vi "Add PV (NT Enum (Enum)).vi"(6 "initial timestamp":timestamp, 7 "PV name":string, 8 "error in (no error)":errorcluster, 10 "initial value":variant, 11 "Server in":refnum<class "Server.lvclass">) -> (0 "error out":errorcluster, 2 "value out":variant, 3 "Server out":refnum<class "Server.lvclass">, 4 "timestamp out":timestamp)   [LabVIEW 2020, in "PV Access.lvlib" / "PVA Server.lvlib" / "Server.lvclass"]
uses:
  Server.lvclass
  PV Data/NT Enum/NT Enum.lvclass
  C:/Users/eyw68381/source/repos/pvaccess-labview/labview/source/PV Data/NT Base/NT Base.lvclass
  <vilib>/Utility/error.llb/Error Cluster From Error Code.vi
  <vilib>/ErrorRing/Error Ring.xnode
  Source/Source.lvclass
  PV Data/PV Data.lvlib
  <userlib>/_OpenG.lib/lvdata/lvdata.llb/openg_variant.lvlib
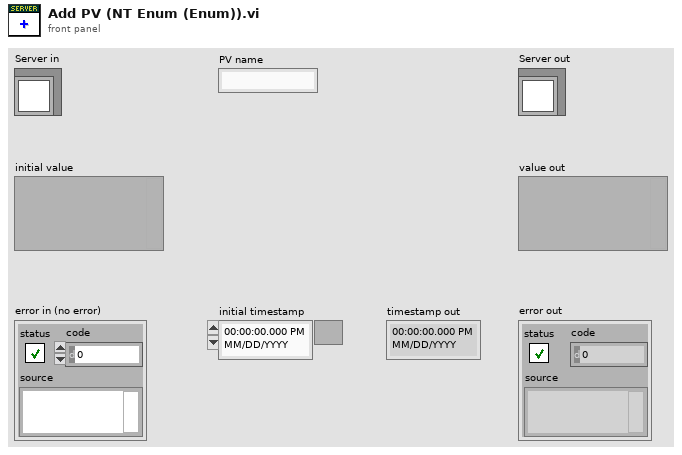
[diagram p1: front panel]
types:
  T1 = typedef "openg_variant.lvlib/Type Descriptor Enumeration__ogtk.ctl" = enum8{"<Null>", "I8", "I16", "I32", "I64", "U8", "U16", "U32", "U64", "SGL", "DBL", "EXT", "CSG", "CDB", "CXT", "0x0F", "0x10", "0x11", "0x12", "0x13", "0x14", "Enum U8", "Enum U16", "Enum U32", "Enum U64", "SGL PQ", "DBL PQ", "EXT PQ", "CSG PQ", "CDB PQ", "CXT PQ", "0x1F", "0x20", "Boolean", "0x22", "0x23", "0x24", "0x25", "0x26", "0x27", "0x28", "0x29", "0x2A", "0x2B", "0x2C", "0x2D", "0x2E", "0x2F", "String", "0x31", "Path", "Pict", "0x34", "0x35", "0x36", "DAQ", "0x38", "0x39", "0x3A", "0x3B", "0x3C", "0x3D", "0x3E", "0x3F", "Array", "0x41", "0x42", "0x43", "0x44", "0x45", "0x46", "0x47", "0x48", "0x49", "0x4A", "0x4B", "0x4C", "0x4D", "0x4E", "0x4F", "Cluster", "0x51", "0x52", "Variant", "Waveform", "0x55", "0x56", "0x57", "0x58", "0x59", "0x5A", "0x5B", "0x5C", "0x5D", "0x5E", "Fixed Point", "0x60", "0x61", "0x62", "0x63", "0x64", "0x65", "0x66", "0x67", "0x68", "0x69", "0x6A", "0x6B", "0x6C", "0x6D", "0x6E", "0x6F", "Refnum", "0x71", "0x72", "Set Collection", "Map Collection"}
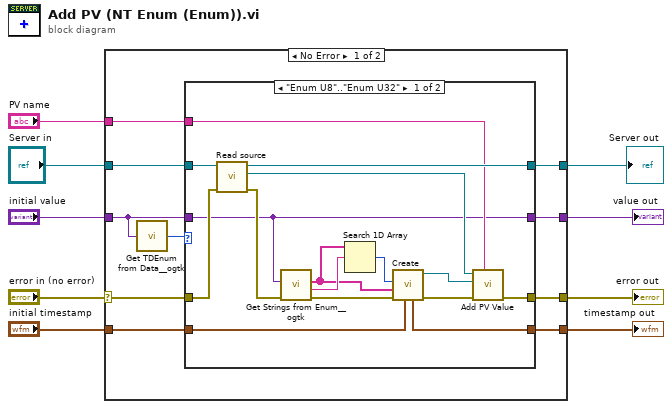
[diagram p0: block diagram]
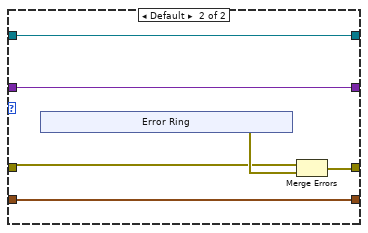
[diagram p2: hidden frame]
diagram:
  n1 = case shown="No Error" "error in (no error)" {
    selector: "error in (no error)" -> [w16 w49]
    tunnel: [w15 w49] -> w9
    tunnel: [w18 w48] -> w7
    tunnel: "Server in" -> [w19 w48]
    tunnel: "PV name" -> [w17 _]
    tunnel: "initial value" -> [w11 w47]
    tunnel: [w10 w47] -> w4
    tunnel: "initial timestamp" -> [w14 w46]
    tunnel: [w13 w46] -> w2
    frame No Error {
      n2 = call <userlib>:"Get TDEnum from Data__ogtk.vi"("Data"=w11) -> ("Type Descriptor Enumeration"=w12:T1)  [unwired: 4 in]
      n3 = case shown="\"Enum U8\"..\"Enum U32\"" w12 {
        tunnel: w19 -> [w35 w37]
        tunnel: [w34 w37] -> w18
        tunnel: w17 -> [w32 _]
        tunnel: w16 -> [w31 w39]
        tunnel: [w30 w38] -> w15
        tunnel: w14 -> [w27 w41]
        tunnel: [w26 w41] -> w13
        tunnel: w11 -> [w20 w36]
        tunnel: [w20 w36] -> w10
        frame "Enum U8".."Enum U32" {
          n4 = call "Read source.vi"("error in (no error)"=w31, "Server in"=w35) -> ("error out"=w23:errorcluster, "Source"=w33:refnum<class "Source.lvclass">, "Server out"=w34:refnum<class "Server.lvclass">)  [unwired: 7 in]
          n5 = call <userlib>:"Get Strings from Enum__ogtk.vi"("error in (no error)"=w23, "Enum"=w20) -> ("error out"=w25:errorcluster, "String Value"=w22:string, "Enum Strings"=w21:string[])  [unwired: 6 in, 1 out]
          n6 = Search 1D Array(1D array=w21, element=w22) -> (index of element=w24:i32)  [unwired: 1 in]
          n7 = call-poly "Create.vi"("initial timestamp"=w27, "error in (no error)"=w25, "choices"=w21, "initial index"=w24) -> ("error out"=w29:errorcluster, "NT Enum out"=w28:refnum<class "NT Enum.lvclass">, "timestamp out"=w26:timestamp)  [unwired: 3 in, 2 out]
          n8 = call "Add PV Value.vi"("PV name"=w32, "error in"=w29, "NT Base in"=w28, "Source in"=w33) -> ("error out"=w30:errorcluster)  [unwired: 5 in, 2 out]
        }
        frame Default {
          n9 = xnode "Error Ring"() -> ("error out"=w40:errorcluster)
          n10 = Merge Errors(w39, w40) -> (w38:errorcluster)
        }
      }
    }
    frame Error {
    }
  }
  "error out" <- w9
  "Server out" <- w7
  "value out" <- w4
  "timestamp out" <- w2
